vi "Counter.vi"() -> ()   [LabVIEW 2017]
uses:
  <vilib>/addons/database/Connection.llb/DB Tools Open Connec (String).vi
  Global/Global 1.vi
  <userlib>/_OpenG.lib/array/array.llb/Empty 2D Array (Variant)__ogtk.vi
  <vilib>/addons/database/NI_Database_API.lvlib
panel:
  in  "CREATE":bool
  in  "Reset Square":bool
  in  "RECIPE NAME":string
  out "RUNNING LOADED RECIPE":string
  in  "BARCODE RECIPE":string(combo)
  in  "Delete Square":bool
  in  "Save Square":bool
  in  "OK2":bool
  in  "FROM":timestamp format="%<%x>T"
  out "error out":errorcluster
  in  "error in (no error)":errorcluster
  in  "EXIT":bool
  in  "SHIFT":string(combo)
  in  "TO":timestamp format="%<%x>T"
  out "OK":i32
  out "TOTAL":i32
  out "NOK":i32
  # "COUNTER"
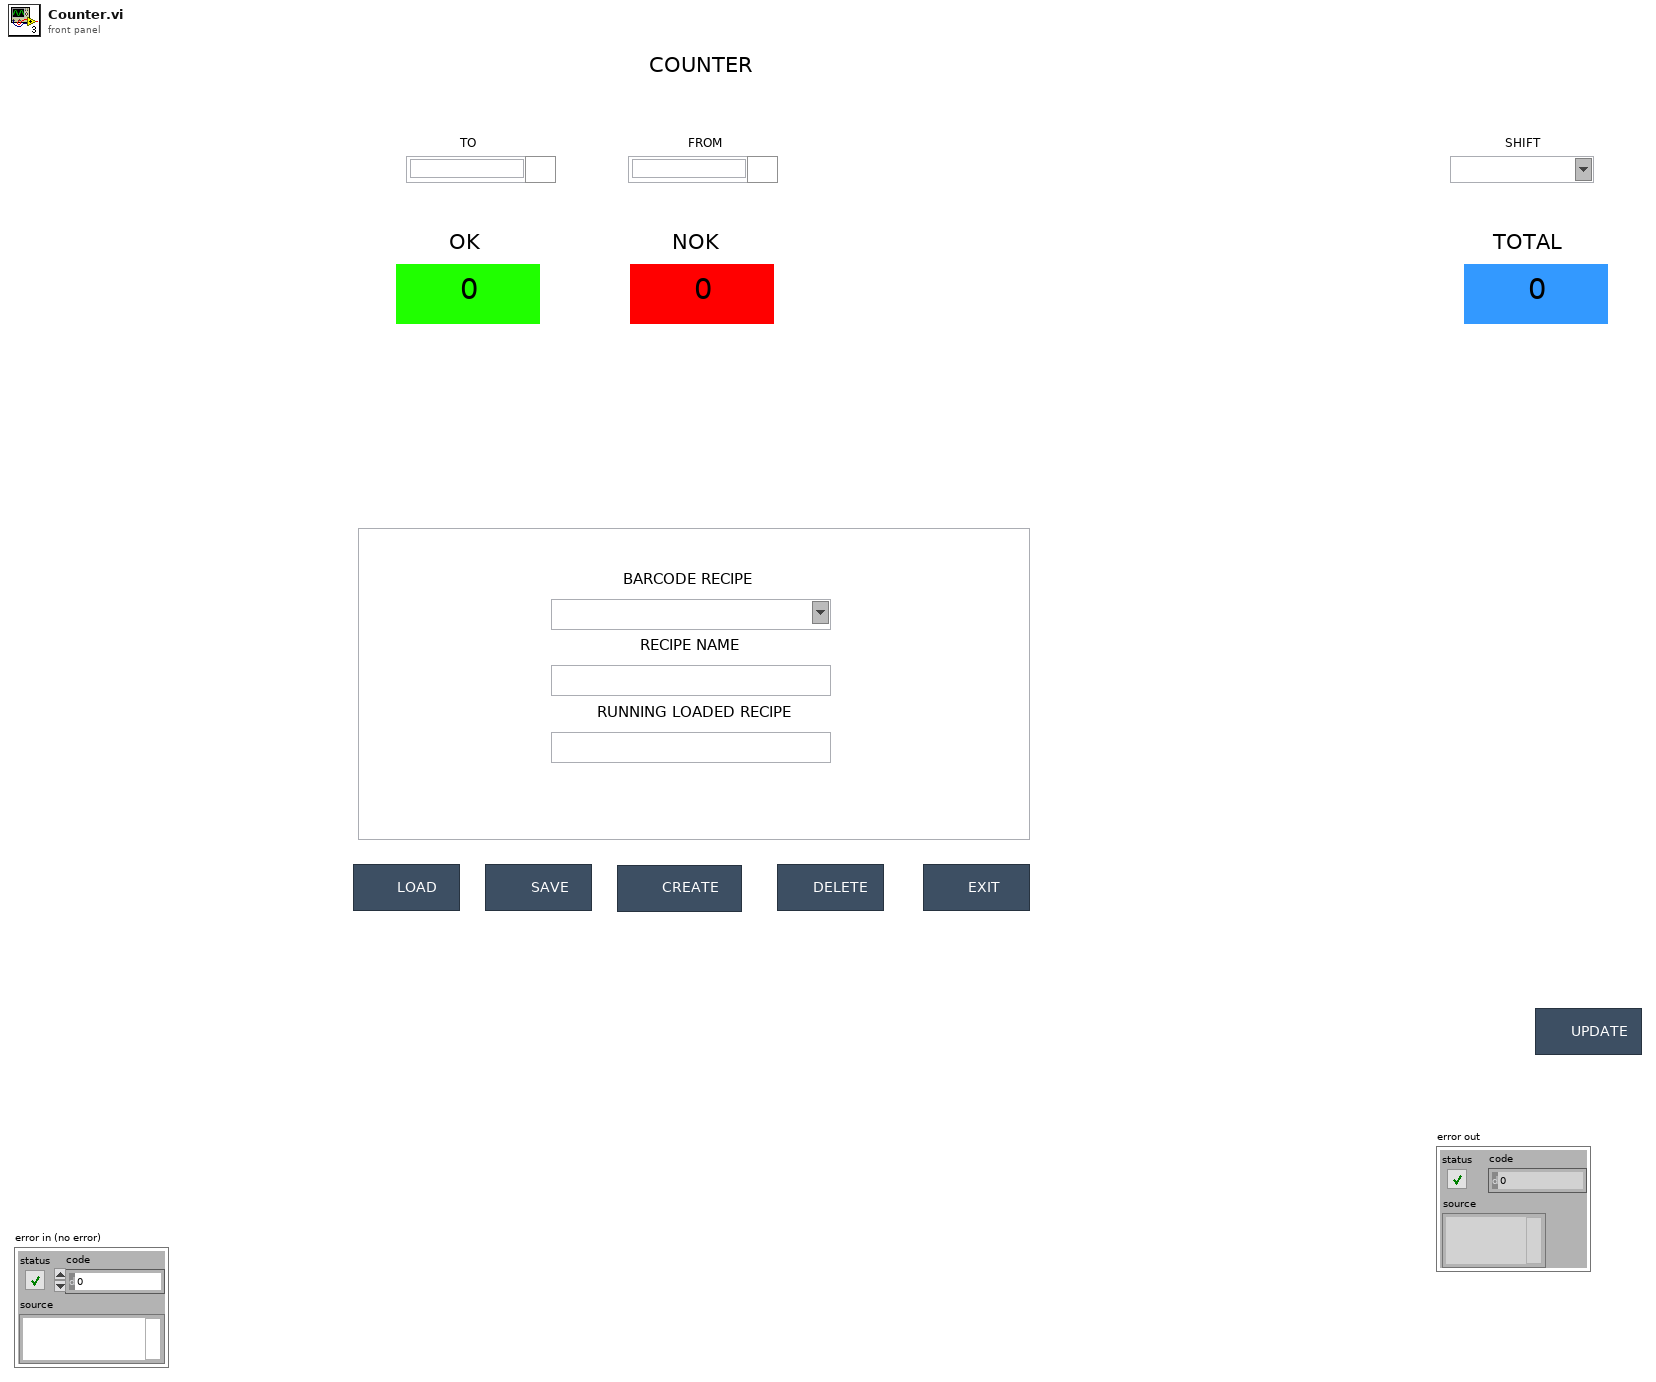
[diagram p1: front panel]
types:
  T1 = typedef "NI_Database_API.lvlib/Conn ObjectReference.ctl" = refnum<k1>
  T2 = cluster{" BARCODE RECIPE":string, "RECIPE NAME":string}
  T3 = enum32{"invalid app kind", "Development System", "Run Time System", "Student Edition", "Embedded LabVIEW", "Evaluation", "Custom"}
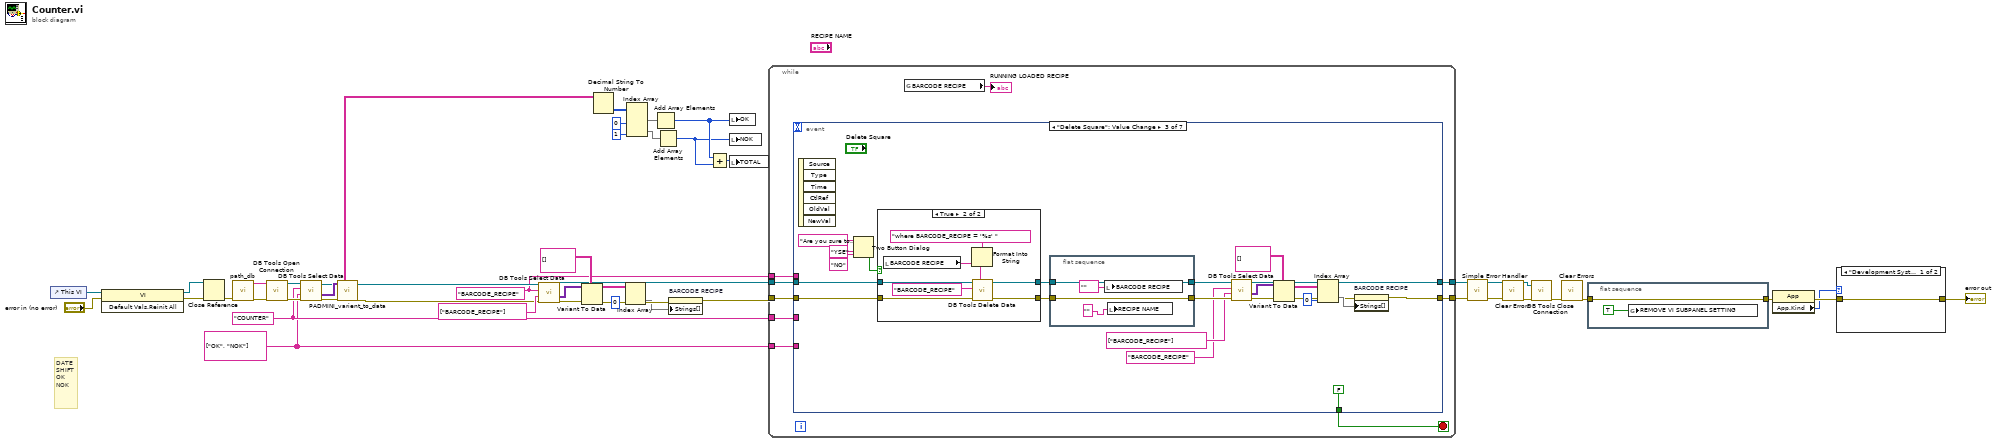
[diagram p0: block diagram]
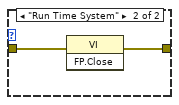
[diagram p2: hidden frame]
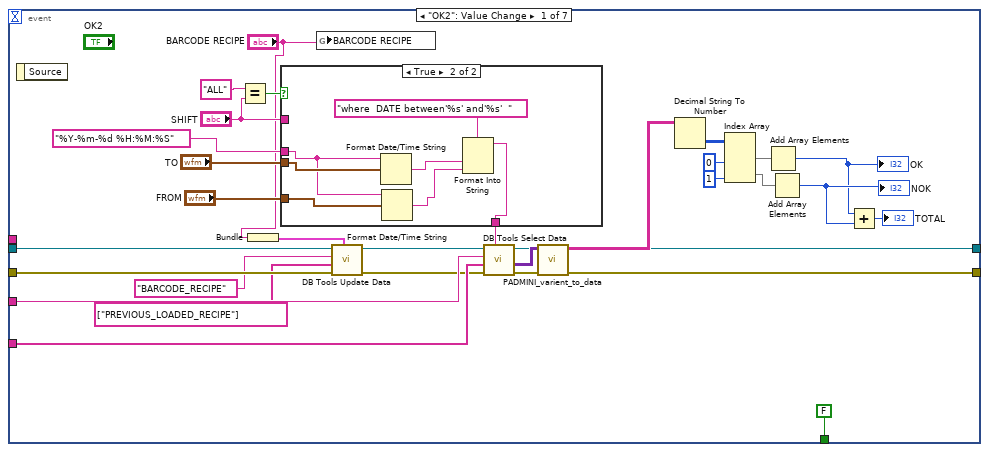
[diagram p3: hidden frame]
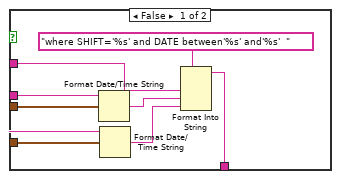
[diagram p4: hidden frame]
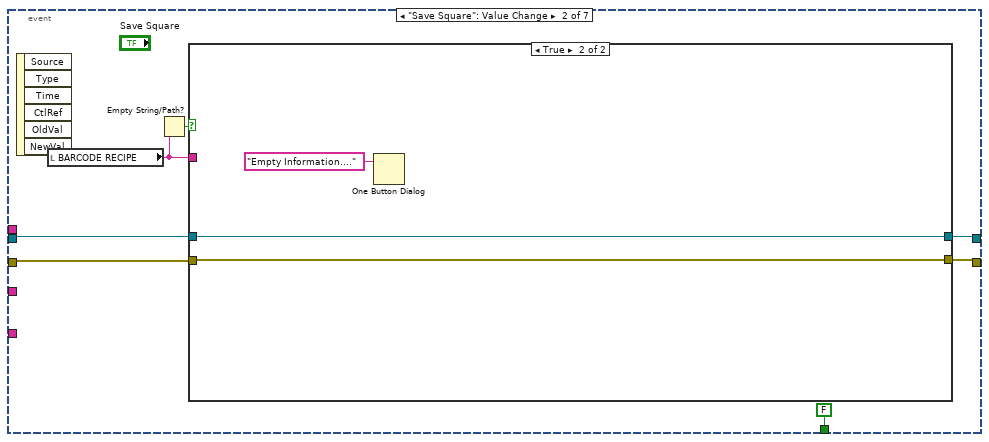
[diagram p5: hidden frame]
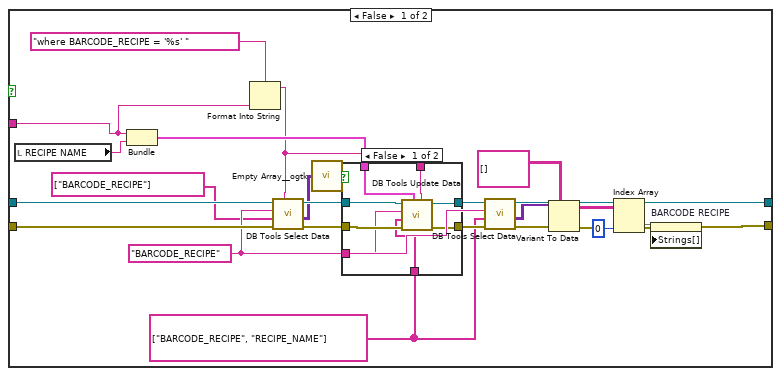
[diagram p6: hidden frame]
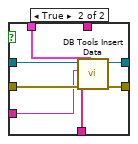
[diagram p7: hidden frame]
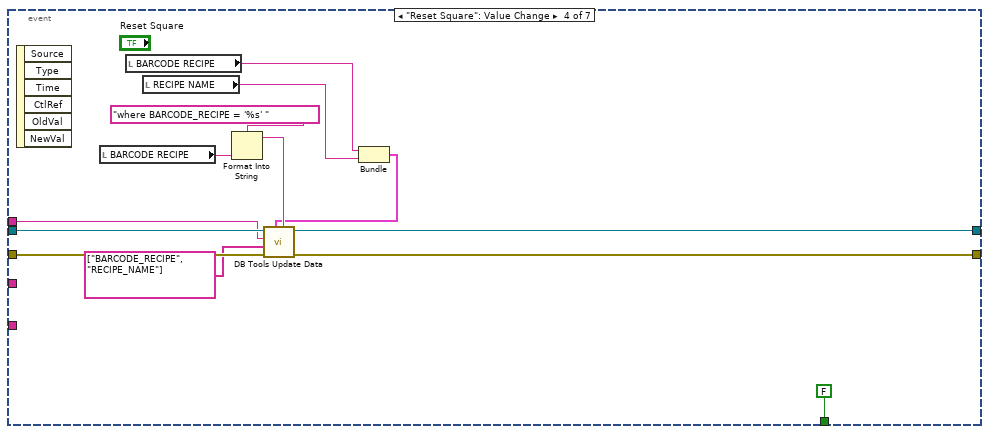
[diagram p9: hidden frame]
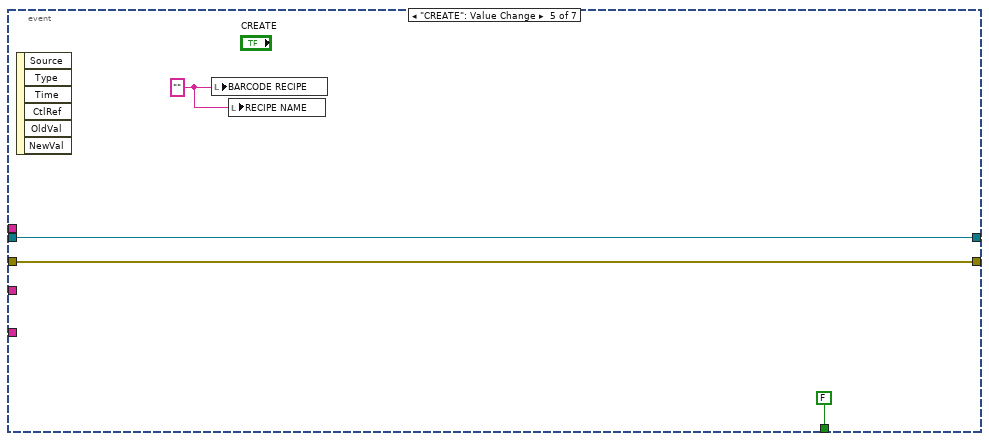
[diagram p10: hidden frame]
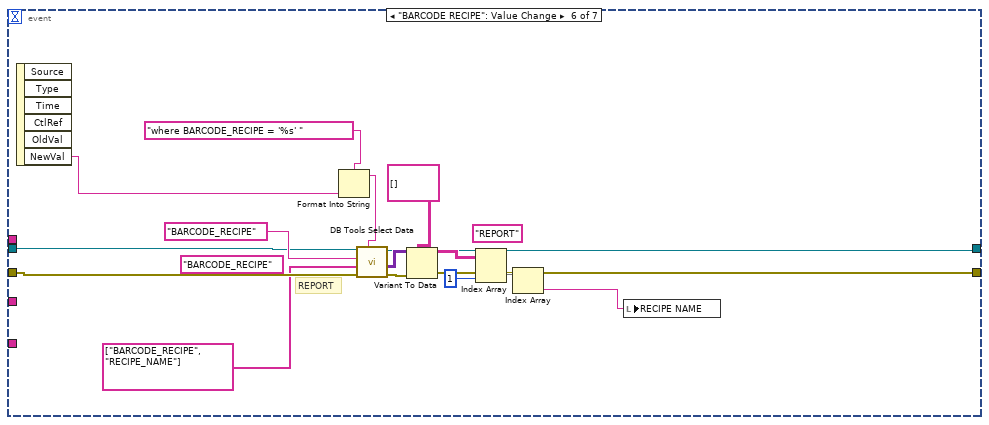
[diagram p11: hidden frame]
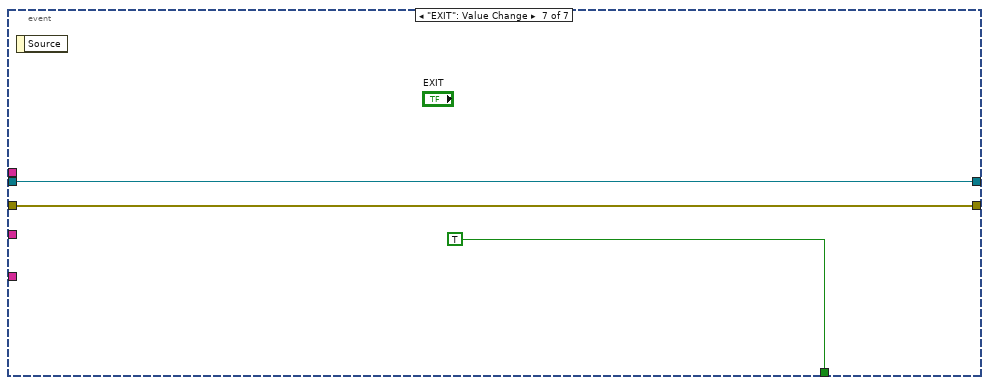
[diagram p12: hidden frame]
diagram:
  w1 = "BARCODE_RECIPE" ("table")
  w14 = string[] ["OK", "NOK"]
  w15 = "COUNTER"
  # "DATE\nSHIFT\nOK\nNOK"
  n1 = control-ref of="This VI"() -> (w43:refnum<vi>)
  n2 = invoke class="VI" method="Default Vals.Reinit All"(reference=w43, error in="error in (no error)") -> (reference out=w41:refnum<vi>, error out=w40:errorcluster)  [unwired: 1 in, 1 out]
  n3 = Close Reference(reference=w41, error in (no error)=w40) -> (error out=w39:errorcluster)
  n4 = call "path_db.vi"("error in"=w39) -> ("error out"=w45:errorcluster, "resulting string"=w44:string)  [unwired: 9 in]
  n5 = call-poly <vilib>:"DB Tools Open Connection.vi"("error in (no error)"=w45, "connection information"=w44) -> ("error out"=w26:errorcluster, "connection reference"=w38:T1)  [unwired: 6 in]
  n6 = call <vilib>:"DB Tools Select Data.vi"("error in (no error)"=w26, "columns"=w14, "table"=w15, "connection reference"=w38) -> ("error out"=w25:errorcluster, "data"=w27:variant[][], "connection reference out"=w4:T1)  [unwired: 2 in]
  n7 = call "PADMINI_varient_to_data.vi"("error in (no error)"=w25, "data"=w27) -> ("error out"=w2:errorcluster, "Array"=w24:string[][])  [unwired: 8 in]
  n8 = call <vilib>:"DB Tools Select Data.vi"("error in (no error)"=w2, "columns"=string[] ["BARCODE_RECIPE"], "table"=w1, "connection reference"=w4) -> ("error out"=w11:errorcluster, "data"=w7:variant[][], "connection reference out"=w5:T1)  [unwired: 2 in]
  n9 = Variant To Data(error in=w11, type=string[][] [], Variant=w7) -> (data=w6:string[][], error out=w13:errorcluster)
  n10 = Decimal String To Number(string=w24) -> (number=w23:i32[][])  [unwired: 2 in, 1 out]
  n11 = Index Array(array=w6, index (col)=0 ("disabled index (col)")) -> (element=w9:string[])  [unwired: 1 in]
  n12 = Index Array(array=w23, index (col) #1=0 ("disabled index (col)"), index (col) #2=1 ("index (col)")) -> (element #1=w20:i32[], element #2=w19:i32[])  [unwired: 2 in]
  n13 = Add Array Elements(numeric array=w20) -> (sum=w18:i32)
  n14 = Add Array Elements(numeric array=w19) -> (sum=w17:i32)
  n15 = property on="BARCODE RECIPE" class="CmbBox"(error in=w13, "Strings[]"=w9) -> (error out=w10:errorcluster)  [unwired: 1 in, 1 out]
  n16 = Add(x=w18, y=w17) -> (x+y=w16:i32)
  n17 = local write "OK"(w18) -> ()
  n18 = local write "NOK"(w17) -> ()
  n19 = local write "TOTAL"(w16) -> ()
  n20 = while {
    tunnel: w10 -> [w53]
    tunnel: w5 -> [w52]
    tunnel: [w51] -> w29
    tunnel: [w50] -> w28
    tunnel: w15 -> [w49]
    tunnel: w14 -> [w48]
    tunnel: w1 -> [w46]
    stop <- w54 stop-if-true
    n21 = event shown="[2] \"Delete Square\": Value Change" {
      selector: _ -> [_ _ _ _ _ _ _]
      dyn-events: _ -> [_ _ _ _ _ _ _]
      timeout: _ -> [_ _ _ _ _ _ _]
      tunnel: [FALSE FALSE FALSE FALSE FALSE _ TRUE] -> w54
      tunnel: w53 -> [w60 w104 w171 w198 w202 w212 w220]
      tunnel: w52 -> [w62 w103 w172 w199 w203 w213 w221]
      tunnel: [w76 w106 w159 w197 w203 w206 w221] -> w51
      tunnel: [w77 w105 w158 w196 w202 w205 w220] -> w50
      tunnel: w49 -> [w75 _ _ _ _ _ _]
      tunnel: w48 -> [w74 _ _ _ _ _ _]
      tunnel: w46 -> [_ _ _ w195 _ _ _]
      event "OK2": Value Change {
        n22 = event-data() -> ()  [unwired: 1 in, 1 out]
        n23 = Equal?(x="ALL", y="SHIFT") -> (x = y?=w65:bool)
        n24 = Bundle("BARCODE RECIPE"="BARCODE RECIPE") -> (w55:cluster{" BARCODE RECIPE":string})  [unwired: 1 in]
        n25 = case shown="True" w65 {
          tunnel: [w93 w95] -> w70
          tunnel: "SHIFT" -> [w91 _]
          tunnel: "TO" -> [w90 w99]
          tunnel: "FROM" -> [w88 w97]
          tunnel: "%Y-%m-%d %H:%M:%S" ("time format string (%c)") -> [w86 w98]
          frame False {
            n26 = Format Date/Time String(time format string (%c)=w86, seconds (now)=w90) -> (date/time string=w89:string)  [unwired: 1 in]
            n27 = Format Date/Time String(time format string (%c)=w86, seconds (now)=w88) -> (date/time string=w87:string)  [unwired: 1 in]
            n28 = Format Into String(format string="where SHIFT='%s' and DATE between'%s' and'%s'  ", w91, w89, w87) -> (resulting string=w93:string)  [unwired: 2 in, 1 out]
          }
          frame True {
            n29 = Format Date/Time String(time format string (%c)=w98, seconds (now)=w99) -> (date/time string=w100:string)  [unwired: 1 in]
            n30 = Format Date/Time String(time format string (%c)=w98, seconds (now)=w97) -> (date/time string=w96:string)  [unwired: 1 in]
            n31 = Format Into String(format string="where  DATE between'%s' and'%s'  ", w100, w96) -> (resulting string=w95:string)  [unwired: 2 in, 1 out]
          }
        }
        n32 = global write "Global 1.vi" "BARCODE RECIPE"("BARCODE RECIPE") -> ()
        n33 = call <vilib>:"DB Tools Update Data.vi"("data"=w55, "error in (no error)"=w60, "columns"=string[] ["PREVIOUS_LOADED_RECIPE"], "table"="BARCODE_RECIPE", "connection reference"=w62) -> ("error out"=w59:errorcluster, "connection reference out"=w61:T1)  [unwired: 5 in]
        n34 = call <vilib>:"DB Tools Select Data.vi"("condition"=w70, "error in (no error)"=w59, "columns"=w74, "table"=w75, "connection reference"=w61) -> ("error out"=w78:errorcluster, "data"=w85:variant[][], "connection reference out"=w76:T1)  [unwired: 1 in]
        n35 = call "PADMINI_varient_to_data.vi"("error in (no error)"=w78, "data"=w85) -> ("error out"=w77:errorcluster, "Array"=w84:string[][])  [unwired: 8 in]
        n36 = Decimal String To Number(string=w84) -> (number=w83:i32[][])  [unwired: 2 in, 1 out]
        n37 = Index Array(array=w83, index (col) #1=0 ("disabled index (col)"), index (col) #2=1 ("index (col)")) -> (element #1=w80:i32[], element #2=w79:i32[])  [unwired: 2 in]
        n38 = Add Array Elements(numeric array=w80) -> (sum=w71:i32)
        "OK" <- w71
        n39 = Add Array Elements(numeric array=w79) -> (sum=w72:i32)
        "NOK" <- w72
        n40 = Add(x=w71, y=w72) -> (x+y=→"TOTAL":i32)
      }
      event "Save Square": Value Change {
        n41 = event-data() -> ()  [unwired: 1 in, 6 out]
        n42 = local read "BARCODE RECIPE"() -> (w101:string)
        n43 = Empty String/Path?(string/path=w101) -> (empty?=w102:bool)
        n44 = case shown="True" w102 {
          tunnel: [w128 w149] -> w106
          tunnel: [w121 w148] -> w105
          tunnel: w104 -> [w118 w148]
          tunnel: w103 -> [w116 w149]
          tunnel: w101 -> [w111 _]
          frame False {
            w120 = string[] ["BARCODE_RECIPE", "RECIPE_NAME"] ("columns")
            w114 = "BARCODE_RECIPE" ("table")
            n45 = local read "RECIPE NAME"() -> (w119:string)
            n46 = Bundle("BARCODE RECIPE"=w111, "RECIPE NAME"=w119) -> (w132:T2)  [unwired: 1 in]
            n47 = Format Into String(format string="where BARCODE_RECIPE = '%s' ", w111) -> (resulting string=w109:string)  [unwired: 2 in, 1 out]
            n48 = call <vilib>:"DB Tools Select Data.vi"("condition"=w109, "error in (no error)"=w118, "columns"=string[] ["BARCODE_RECIPE"] ("String"), "table"=w114, "connection reference"=w116) -> ("error out"=w117:errorcluster, "data"=w110:variant[][], "connection reference out"=w115:T1)  [unwired: 1 in]
            n49 = call-poly <userlib>:"Empty Array__ogtk.vi"("Array"=w110) -> ("Empty Array?"=w108:bool)  [unwired: 8 in]
            n50 = case shown="False" w108 {
              tunnel: w117 -> [w139 w147]
              tunnel: w115 -> [w140 w146]
              tunnel: w132 -> [w135 w145]
              tunnel: [w138 w144] -> w131
              tunnel: [w137 w143] -> w129
              tunnel: w114 -> [w133 w142]
              tunnel: w120 -> [w134 w141]
              tunnel: w109 -> [w136 _]
              frame False {
                n51 = call <vilib>:"DB Tools Update Data.vi"("condition"=w136, "data"=w135, "error in (no error)"=w139, "columns"=w134, "table"=w133, "connection reference"=w140) -> ("error out"=w138:errorcluster, "connection reference out"=w137:T1)  [unwired: 4 in]
              }
              frame True {
                n52 = call <vilib>:"DB Tools Insert Data.vi"("data"=w145, "error in (no error)"=w147, "columns"=w141, "table"=w142, "connection reference"=w146) -> ("error out"=w144:errorcluster, "connection reference out"=w143:T1)  [unwired: 5 in]
              }
            }
            n53 = call <vilib>:"DB Tools Select Data.vi"("error in (no error)"=w131, "columns"=w120, "table"=w114, "connection reference"=w129) -> ("error out"=w130:errorcluster, "data"=w126:variant[][], "connection reference out"=w128:T1)  [unwired: 2 in]
            n54 = Variant To Data(error in=w130, type=string[][] [], Variant=w126) -> (data=w125:string[][], error out=w122:errorcluster)
            n55 = Index Array(array=w125, index (col)=0 ("disabled index (col)")) -> (element=w123:string[])  [unwired: 1 in]
            n56 = property on="BARCODE RECIPE" class="CmbBox"(error in=w122, "Strings[]"=w123) -> (error out=w121:errorcluster)  [unwired: 1 in, 1 out]
          }
          frame True {
            n57 = One Button Dialog(message="Empty Information....") -> ()  [unwired: 1 in, 1 out]
          }
        }
      }
      event "Delete Square": Value Change {
        n58 = event-data() -> ()  [unwired: 1 in, 6 out]
        n59 = Two Button Dialog(message="Are you sure to want delete this barcode recipe?", 1:"NO" ("F button name (\"Cancel\")"), 2:"YSE" ("T button name (\"OK\")")) -> (T button?=w152:bool)
        n60 = case shown="True" w152 {
          tunnel: w172 -> [w174 w182]
          tunnel: w171 -> [w173 w181]
          tunnel: [w173 w177] -> w170
          tunnel: [w174 w176] -> w169
          frame False {
          }
          frame True {
            n61 = local read "BARCODE RECIPE"() -> (w179:string)
            n62 = Format Into String(format string="where BARCODE_RECIPE = '%s' ", w179) -> (resulting string=w178:string)  [unwired: 2 in, 1 out]
            n63 = call <vilib>:"DB Tools Delete Data.vi"("condition"=w178, "error in (no error)"=w181, "table"="BARCODE_RECIPE", "connection reference"=w182) -> ("error out"=w177:errorcluster, "connection reference out"=w176:T1)  [unwired: 6 in]
          }
        }
        n64 = flat-sequence {
          tunnel: [w186] -> w160
          tunnel: w170 -> [w186]
          tunnel: [w184] -> w161
          tunnel: w169 -> [w184]
          frame #0 {
            n65 = local write "BARCODE RECIPE"("" ("BARCODE RECIPE")) -> ()
            n66 = local write "RECIPE NAME"("") -> ()
          }
        }
        n67 = call <vilib>:"DB Tools Select Data.vi"("error in (no error)"=w160, "columns"=string[] ["BARCODE_RECIPE"], "table"="BARCODE_RECIPE", "connection reference"=w161) -> ("error out"=w168:errorcluster, "data"=w167:variant[][], "connection reference out"=w159:T1)  [unwired: 2 in]
        n68 = Variant To Data(error in=w168, type=string[][] [], Variant=w167) -> (data=w166:string[][], error out=w164:errorcluster)
        n69 = Index Array(array=w166, index (col)=0 ("disabled index (col)")) -> (element=w165:string[])  [unwired: 1 in]
        n70 = property on="BARCODE RECIPE" class="CmbBox"(error in=w164, "Strings[]"=w165) -> (error out=w158:errorcluster)  [unwired: 1 in, 1 out]
      }
      event "Reset Square": Value Change {
        n71 = event-data() -> ()  [unwired: 1 in, 6 out]
        n72 = local read "BARCODE RECIPE"() -> (w193:string)
        n73 = local read "BARCODE RECIPE"() -> (w190:string)
        n74 = local read "RECIPE NAME"() -> (w189:string)
        n75 = Format Into String(format string="where BARCODE_RECIPE = '%s' ", w193) -> (resulting string=w191:string)  [unwired: 2 in, 1 out]
        n76 = Bundle("BARCODE RECIPE"=w190, "RECIPE NAME"=w189) -> (w188:T2)  [unwired: 1 in]
        n77 = call <vilib>:"DB Tools Update Data.vi"("condition"=w191, "data"=w188, "error in (no error)"=w198, "columns"=string[] ["BARCODE_RECIPE", "RECIPE_NAME"], "table"=w195, "connection reference"=w199) -> ("error out"=w196:errorcluster, "connection reference out"=w197:T1)  [unwired: 4 in]
      }
      event "CREATE": Value Change {
        w200 = ""
        n78 = event-data() -> ()  [unwired: 1 in, 6 out]
        n79 = local write "BARCODE RECIPE"(w200) -> ()
        n80 = local write "RECIPE NAME"(w200) -> ()
      }
      event "BARCODE RECIPE": Value Change {
        (unwired) "BARCODE_RECIPE" ("String")
        (unwired) "REPORT"
        # "REPORT"
        n81 = event-data() -> ("NewVal"=w209:string)  [unwired: 1 in, 5 out]
        n82 = Format Into String(format string="where BARCODE_RECIPE = '%s' ", w209) -> (resulting string=w210:string)  [unwired: 2 in, 1 out]
        n83 = call <vilib>:"DB Tools Select Data.vi"("condition"=w210, "error in (no error)"=w212, "columns"=string[] ["BARCODE_RECIPE", "RECIPE_NAME"], "table"="BARCODE_RECIPE", "connection reference"=w213) -> ("error out"=w218:errorcluster, "data"=w217:variant[][], "connection reference out"=w206:T1)  [unwired: 1 in]
        n84 = Variant To Data(error in=w218, type=string[][] [], Variant=w217) -> (data=w216:string[][], error out=w205:errorcluster)
        n85 = Index Array(array=w216, index (col)=1 ("disabled index (col)")) -> (element=w214:string[])  [unwired: 1 in]
        n86 = Index Array(array=w214) -> (element=w204:string)  [unwired: 1 in]
        n87 = local write "RECIPE NAME"(w204) -> ()
      }
      event "EXIT": Value Change {
        n88 = event-data() -> ()  [unwired: 1 in, 1 out]
      }
    }
    n89 = global read "Global 1.vi" "BARCODE RECIPE"() -> (→"RUNNING LOADED RECIPE":string)
  }
  n90 = call <vilib>:"Simple Error Handler.vi"("error in (no error)"=w28) -> ("error out"=w35:errorcluster)  [unwired: 4 in, 4 out]
  n91 = call <vilib>:"Clear Errors.vi"("error in (no error)"=w35) -> ("error out"=w34:errorcluster)  [unwired: 5 in, 1 out]
  n92 = call <vilib>:"DB Tools Close Connection.vi"("error in (no error)"=w34, "connection reference"=w29) -> ("error out"=w37:errorcluster)  [unwired: 5 in]
  n93 = call <vilib>:"Clear Errors.vi"("error in (no error)"=w37) -> ("error out"=w31:errorcluster)  [unwired: 5 in, 1 out]
  n94 = flat-sequence {
    tunnel: w31 -> [w224]
    tunnel: [w224] -> w30
    frame #0 {
      n95 = global write "Global 1.vi" "REMOVE VI SUBPANEL SETTING"(TRUE ("remove_VI")) -> ()
    }
  }
  n96 = property class="App"(error in=w30) -> (error out=w33:errorcluster, "App.Kind"=w32:T3)  [unwired: 1 in, 1 out]
  n97 = case shown="\"Development System\", Default" w32 {
    tunnel: [w225 w227] -> w36
    tunnel: w33 -> [w225 w226]
    frame "Development System", Default {
    }
    frame "Run Time System" {
      n98 = invoke class="VI" method="FP.Close"(error in=w226) -> (error out=w227:errorcluster)  [unwired: 2 in, 2 out]
    }
  }
  "error out" <- w36
